vi "GetNegativeFixInt.vi"(8 "error in (no error)":errorcluster, 11 "MsgPackDeserializer in":refnum<class "MsgPackDeserializer.lvclass">) -> (0 "error out":errorcluster, 2 "Number":u8, 3 "MsgPackDeserializer out":refnum<class "MsgPackDeserializer.lvclass">)   [LabVIEW 2015, in "MsgPackDeserializer.lvclass"]
uses:
  MsgPackDeserializer.lvclass
  MsgPackDeserializer.lvclass/MsgPackDeserializer.ctl
panel:
  out "Boolean array":bool[](array[boolean])
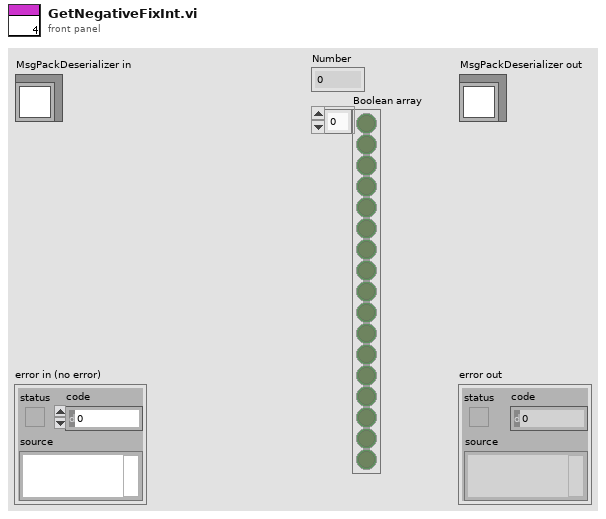
[diagram p1: front panel]
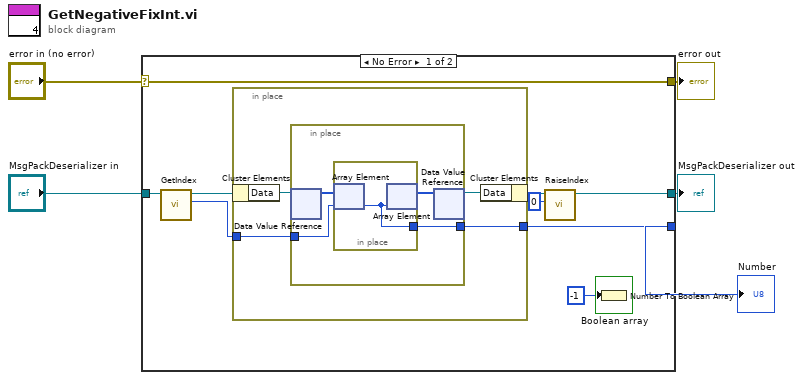
[diagram p0: block diagram]
diagram:
  n1 = case shown="No Error" "error in (no error)" {
    selector: "error in (no error)" -> [w15 w26]
    tunnel: [w15 w26] -> w4
    tunnel: [w11 w25] -> w2
    tunnel: "MsgPackDeserializer in" -> [w14 w25]
    tunnel: [w9 _] -> w1
    frame No Error {
      n2 = call "GetIndex.vi"("MsgPackDeserializer in"=w14) -> ("Index"=w12:i64, "MsgPackDeserializer out"=w13:refnum<class "MsgPackDeserializer.lvclass">)  [unwired: 8 in, 1 out]
      n3 = in-place {
        in-place-border: [w18] -> w9
        in-place-border: w12 -> [w17]
        n4 = in-place-cluster #1(w13) -> ("Data"=w16:refnum<data-value>)
        n5 = in-place {
          in-place-border: [w23] -> w18
          in-place-border: w17 -> [w22]
          n6 = in-place-dvr #2(w16) -> (w21:u8[])  [unwired: 1 out]
          n7 = in-place {
            in-place-border: [w24] -> w23
            n8 = in-place-array #3(w21, w22) -> (w24:u8)
            n9 = in-place-array #3(w24) -> (w20:u8[])  [unwired: 1 out]
          }
          n10 = in-place-dvr #2(w20) -> (w19:refnum<data-value>)  [unwired: 1 out]
        }
        n11 = in-place-cluster #1("Data"=w19) -> (w10:refnum<class "MsgPackDeserializer.lvclass">)
      }
      n12 = call "RaiseIndex.vi"("x"=i64 0, "MsgPackDeserializer in"=w10) -> ("MsgPackDeserializer out"=w11:refnum<class "MsgPackDeserializer.lvclass">)  [unwired: 8 in, 1 out]
      n13 = Number To Boolean Array(number=i8 -1) -> (Boolean array=→"Boolean array":bool[])
    }
    frame Error {
    }
  }
  "error out" <- w4
  "MsgPackDeserializer out" <- w2
  "Number" <- w1
